vi "_005.vi"() -> ()   [LabVIEW 2024]
panel:
  out "Carry :":bool
  out "Sum :":bool
  in  "C in":bool
  in  "B":bool
  in  "A":bool
  out "Carry :":bool
  out "Sum :":bool
  in  "B":bool
  in  "A":bool
  # "Adders :"
  # "Half Adder ( Truth Table ) :"
  # "Inputs      Outputs \nA  B   Sum   Carry \n0  0  -> 0       0 \n0  1   -> 1        0\n1   0  -> 1        0\n1   1   -> 0       1"
  # "Full Adder ( Truth Table ) :"
  # "Inputs      Outputs      \nA  B C in   Sum   Carry \n0  0   0  ->  0       0 \n0  0   1   ->  1        0\n0  1    0  ->  1        0\n0  1    1   ->  0       1\n1   0   0  ->  1        0\n1   0   1   ->  0       1\n1   1    0  ->  0       1\n1   1    1   ->  1        1"
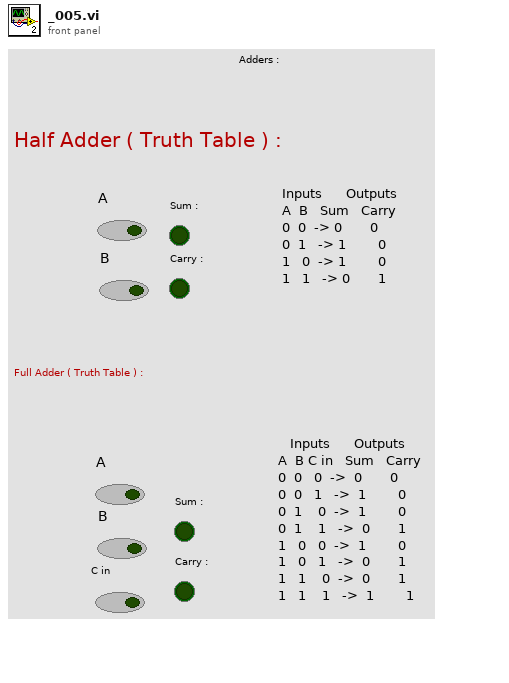
[diagram p1: front panel]
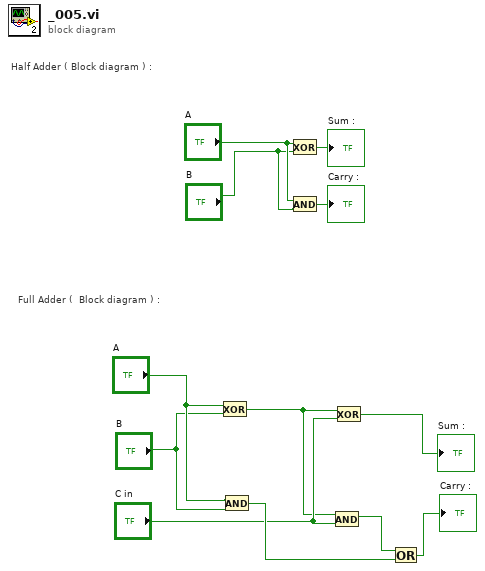
[diagram p0: block diagram]
diagram:
  # "Half Adder ( Block diagram ) :"
  # "Full Adder (  Block diagram ) :"
  n1 = Exclusive Or(1:"B", 2:"A") -> (0:w1:bool)
  n2 = And(x="A", y="B") -> (x .and. y?=w7:bool)
  n3 = Exclusive Or(1:"B", 2:"A") -> (0:→"Sum :":bool)
  n4 = And(x="A", y="B") -> (x .and. y?=→"Carry :":bool)
  n5 = And(x=w1, y="C in") -> (x .and. y?=w6:bool)
  n6 = Exclusive Or(1:"C in", 2:w1) -> (0:→"Sum :":bool)
  n7 = Or(x=w6, y=w7) -> (x .or. y?=→"Carry :":bool)
